vi "SetParam.vi"(8 "error in (no error)":errorcluster caption="entrée d'erreur (pas d'erreur)", 10 "v_measure_score":cluster{"beta":dbl}={"beta"=1.0}, 11 "V_Measure_Score.lvclass":refnum<class "V_Measure_Score.lvclass">) -> (0 "error out":errorcluster caption="sortie d'erreur", 3 "V_Measure_Score.lvclass":refnum<class "V_Measure_Score.lvclass">)   [LabVIEW 2020, in "V_Measure_Score.lvclass"]
doc: "Set Parameters"
uses:
  V_Measure_Score.lvclass
  V_Measure_Score.lvclass/V_Measure_Score.ctl
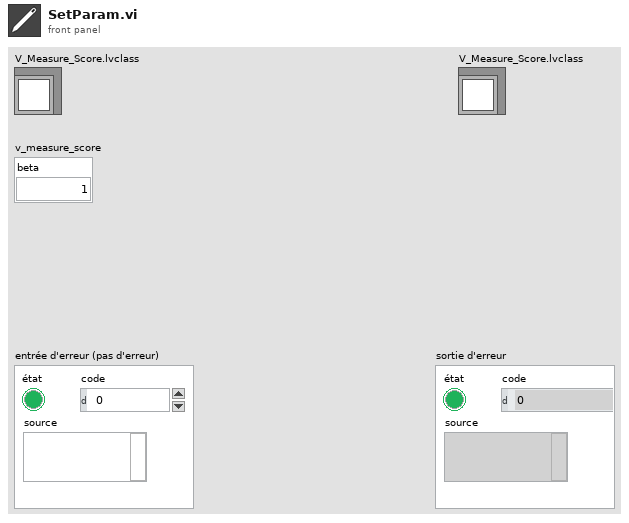
[diagram p1: front panel]
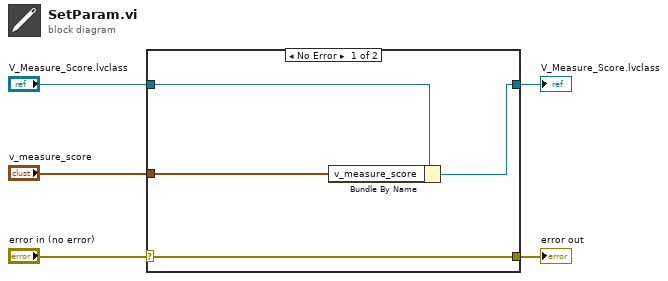
[diagram p0: block diagram]
diagram:
  n1 = case shown="No Error" "error in (no error)" {
    selector: "error in (no error)" -> [w9 w10]
    tunnel: [w9 w10] -> w4
    tunnel: [w7 w11] -> w2
    tunnel: "V_Measure_Score.lvclass" -> [w8 w11]
    tunnel: "v_measure_score" -> [w6 _]
    frame No Error {
      n2 = Bundle By Name(cluster=w8, "v_measure_score"=w6) -> (w7:refnum<class "V_Measure_Score.lvclass">)
    }
    frame Error {
    }
  }
  "error out" <- w4
  "V_Measure_Score.lvclass" <- w2
